vi "read line from internal stream.vi"(8 "error in":errorcluster, 9 "max length":u64, 10 "delimiter":u8=10 format="%.0x", 11 "socket":u64) -> (0 "error out":errorcluster, 3 "buffer":string)   [LabVIEW 2016, in "async tls dl.lvlib"]
uses:
  async tls dl.lvlib
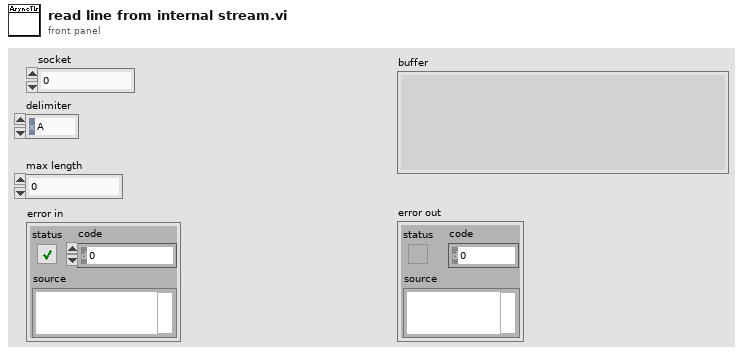
[diagram p1: front panel]
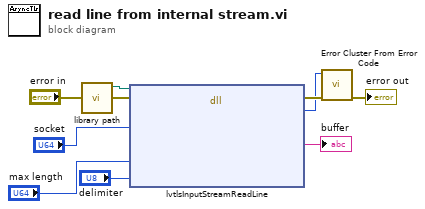
[diagram p0: block diagram]
diagram:
  n1 = call "library path.vi"() -> ("path"=w2:path)  [unwired: 11 in]
  n2 = dll-call lib="C:/Users/IEUser/Desktop/libasynclvtls/lvasynctls.dll" fn="lvtlsInputStreamReadLine" ("lvasynctls.dll:lvtlsInputStreamReadSome")(path in=w2, error in="error in", "socket"="socket", "maxlen"="max length", "delimiter"="delimiter") -> (error out=w9:errorcluster, "err"=w8:i32, "buffer"=→"buffer":string)  [unwired: 5 in, 1 out]
  n3 = call <vilib>:"Error Cluster From Error Code.vi"("error in (no error)"=w9, "error code (0)"=w8) -> ("error out"=→"error out":errorcluster)  [unwired: 7 in]
